vi "GetAvailableCommands.vi"(11 "Select Module":T1) -> (2 "Subdiagram Labels":string[](array[string]), 3 "Available Commands":string[](array[string]))   [LabVIEW 2018]
uses:
  AvailableModules.ctl
  NistPluggableModules/TestClass/Test.lvclass
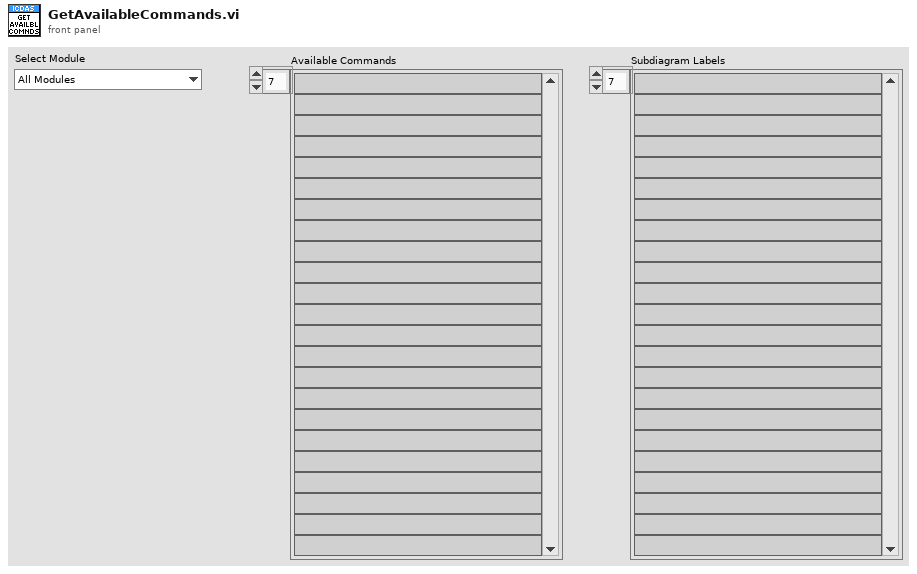
[diagram p1: front panel]
types:
  T1 = typedef "AvailableModules.ctl" = enum16{"All Modules", "AcPwr", "Analysis", "Digitizer", "FGen", "Scope", "Sensor", "Sync"}
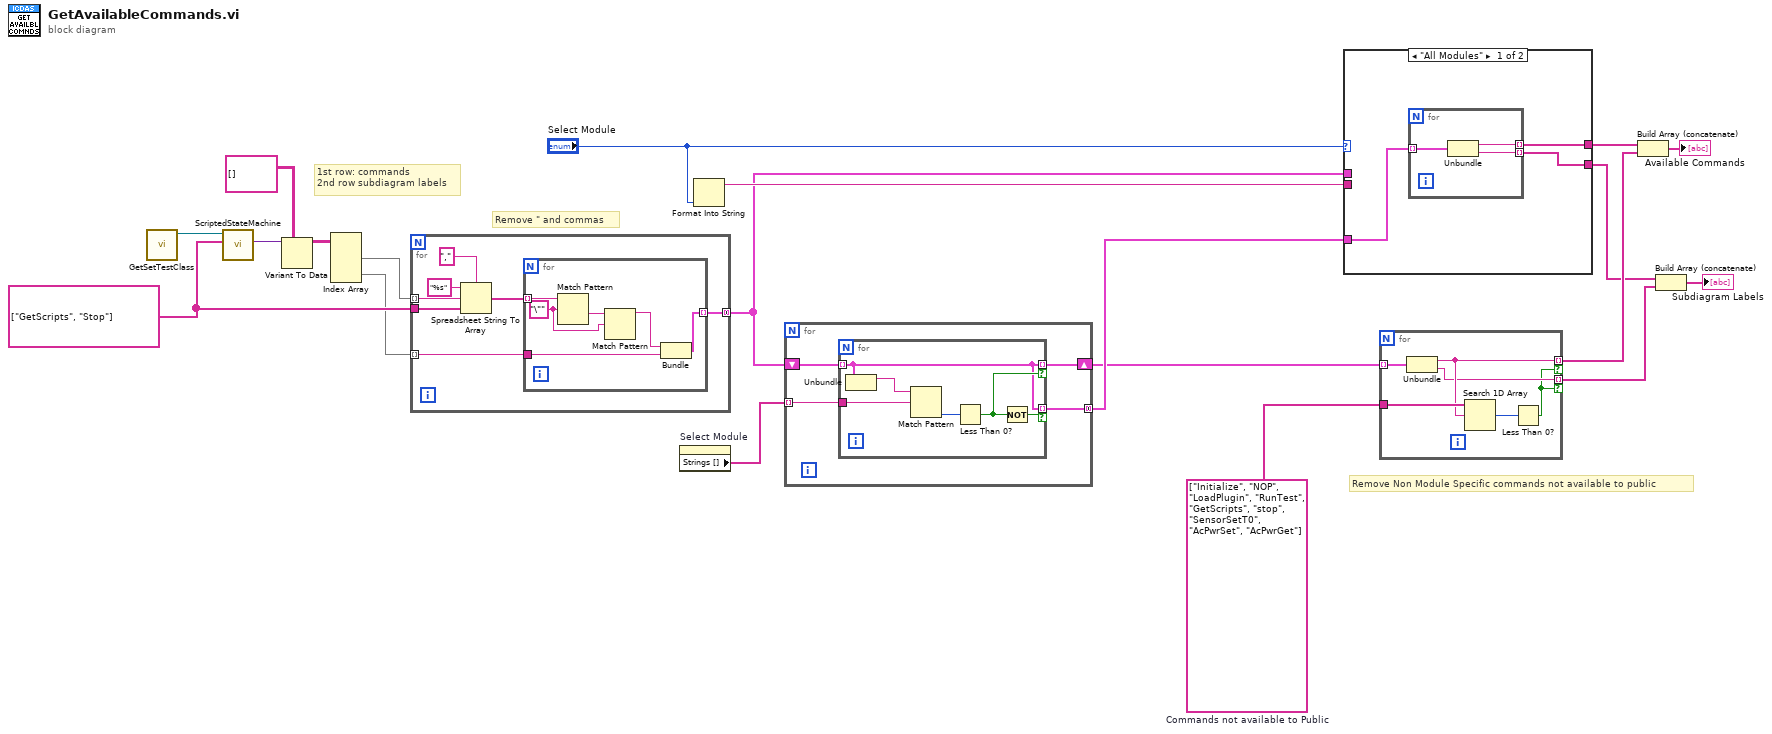
[diagram p0: block diagram]
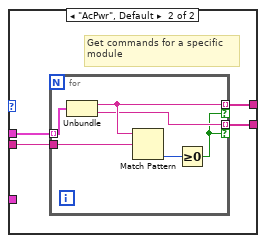
[diagram p2: hidden frame]
diagram:
  w8 = string[] ["GetScripts", "Stop"] ("script")
  w14 = string[] ["Initialize", "NOP", "LoadPlugin", "RunTest", "GetScripts", "stop", "SensorSetT0", "AcPwrSet", "AcPwrGet"]  # Commands not available to Public
  # "1st row: commands\n2nd row subdiagram labels"
  # "Remove Non Module Specific commands not available to public"
  # "Remove \" and commas"
  n1 = call "GetSetTestClass.vi"() -> ("Test.lvclass"=w11:refnum<class "Test.lvclass">)  [unwired: 11 in]
  n2 = call "ScriptedStateMachine.vi"("script"=w8, "Test.lvclass 2"=w11) -> ("Data"=w10:variant)  [unwired: 7 in, 2 out]
  n3 = Variant To Data(type=string[][] [] ("array"), Variant=w10) -> (data=w6:string[][])  [unwired: 1 in, 1 out]
  n4 = Index Array(array=w6) -> (element #1=w5:string[], element #2=w4:string[])  [unwired: 4 in]
  n5 = for {
    tunnel: w5 -> [w26] mode=indexing
    tunnel: w8 -> [w24]
    tunnel: [w22] -> w9 mode=concatenating
    tunnel: w4 -> [w21] mode=indexing
    n6 = Spreadsheet String To Array(delimiter (Tab)=",", format string="%s", spreadsheet string=w26, array type (2D Dbl)=w24) -> (array=w23:string[])
    n7 = for {
      tunnel: w23 -> [w33] mode=indexing
      tunnel: [w28] -> w22 mode=indexing
      tunnel: w21 -> [w30]
      w31 = "\"" ("regular expression")
      n8 = Match Pattern(string=w33, regular expression=w31) -> (after substring=w32:string)  [unwired: 1 in, 3 out]
      n9 = Match Pattern(string=w32, regular expression=w31) -> (before substring=w29:string)  [unwired: 1 in, 3 out]
      n10 = Bundle("String"=w29, "String"=w30) -> (w28:cluster{"String":string, "String":string})  [unwired: 1 in]
    }
  }
  n11 = property on="Select Module" class="Enum (strict)"() -> ("Strings []"=w20:string[])  [unwired: 2 in, 2 out]
  n12 = Format Into String("Select Module") -> (resulting string=w12:string)  [unwired: 3 in, 1 out]
  n13 = for {
    tunnel: w20 -> [w36] mode=indexing
    shift-right: [w34] -> w18
    shift-left: w9 -> [w37]
    tunnel: [w35] -> w19 mode=concatenating
    n14 = for {
      tunnel: w37 -> [w38] mode=indexing
      tunnel: w36 -> [w43]
      tunnel: [w38] -> w34 mode=indexing if=w41
      tunnel: [w38] -> w35 mode=indexing if=w40
      n15 = Unbundle(w38) -> ("String"=w39:string)  [unwired: 1 out]
      n16 = Match Pattern(string=w39, regular expression=w43) -> (offset past match=w42:i32)  [unwired: 1 in, 3 out]
      n17 = Less Than 0?(x=w42) -> (x < 0?=w41:bool)
      n18 = Not(x=w41) -> (.not. x?=w40:bool)
    }
  }
  n19 = case shown="\"All Modules\"" "Select Module" {
    tunnel: w12 -> [_ w53]
    tunnel: w9 -> [_ w52]
    tunnel: [w46 w51] -> w15
    tunnel: w19 -> [w45 _]
    tunnel: [w44 w50] -> w3
    frame "All Modules" {
      n20 = for {
        tunnel: w45 -> [w49] mode=indexing
        tunnel: [w48] -> w46 mode=indexing
        tunnel: [w47] -> w44 mode=indexing
        n21 = Unbundle(w49) -> ("String"=w48:string, "String"=w47:string)
      }
    }
    frame "AcPwr", Default {
      # "Get commands for a specific\nmodule"
      n22 = for {
        tunnel: w52 -> [w57] mode=indexing
        tunnel: w53 -> [w59]
        tunnel: [w56] -> w51 mode=indexing if=w54
        tunnel: [w55] -> w50 mode=indexing if=w54
        n23 = Unbundle(w57) -> ("String"=w56:string, "String"=w55:string)
        n24 = Match Pattern(string=w56, regular expression=w59) -> (offset past match=w58:i32)  [unwired: 1 in, 3 out]
        n25 = Greater Or Equal To 0?(x=w58) -> (x >= 0?=w54:bool)
      }
    }
  }
  n26 = for {
    tunnel: w18 -> [w63] mode=indexing
    tunnel: w14 -> [w64]
    tunnel: [w62] -> w16 mode=indexing if=w60
    tunnel: [w61] -> w2 mode=indexing if=w60
    n27 = Unbundle(w63) -> ("String"=w62:string, "String"=w61:string)
    n28 = Search 1D Array(1D array=w64, element=w62) -> (index of element=w65:i32)  [unwired: 1 in]
    n29 = Less Than 0?(x=w65) -> (x < 0?=w60:bool)
  }
  n30 = Build Array (concatenate)(w15, w16) -> (→"Available Commands":string[])
  n31 = Build Array (concatenate)(w3, w2) -> (→"Subdiagram Labels":string[])
